vi "Data Store.vi"(7 "Store Value CH0":bool, 8 "VDC INPUT2":dbl format="%#.6g", 9 "VDC INPUT1":dbl, 10 "Store Value 2 IN1":bool, 11 "Store Value 1 IN1":bool) -> (2 "Saved Value 2 IN1":dbl, 3 "Saved Value 1 IN1":dbl, 6 "Saved Value CH0":dbl)   [LabVIEW 2012]
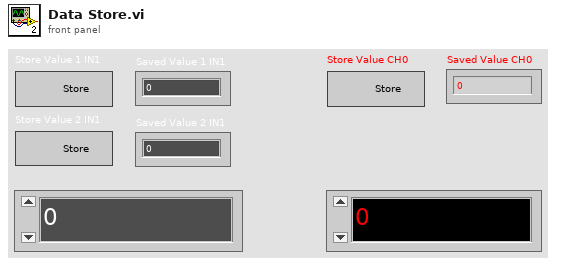
[diagram p1: front panel]
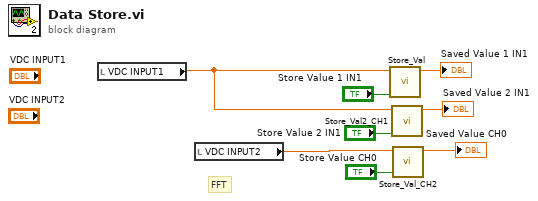
[diagram p0: block diagram]
diagram:
  # "FFT"
  n1 = local read "VDC INPUT1"() -> (w1:dbl)
  n2 = local read "VDC INPUT2"() -> (w2:dbl)
  n3 = call "Store_Val.vi"("Store"="Store Value 1 IN1", "Vin"=w1) -> ("Saved Value"=→"Saved Value 1 IN1":dbl)  [unwired: 9 in]
  n4 = call "Store_Val2_CH1.vi"("Store"="Store Value 2 IN1", "Vin"=w1) -> ("Saved Value"=→"Saved Value 2 IN1":dbl)  [unwired: 9 in]
  n5 = call "Store_Val_CH2.vi"("Store"="Store Value CH0", "Vin"=w2) -> ("Saved Value"=→"Saved Value CH0":dbl)  [unwired: 9 in]
